vi "Load_Waveform.vi"(7 "Cmd":string="CWM", 8 "error in":errorcluster {"code" format="%.0x"}, 11 "RFSG_In":refnum<k15>="VST") -> (0 "error out":errorcluster, 3 "RFSG_Out":refnum<k15>="VST")   [LabVIEW 2014]
uses:
  <vilib>/RF Toolkits/LTE/SG/Support/Includes/nilte toolkit compatibility version.ctl
  <vilib>/RF Toolkits/WCDMA/Generation/Controls/niWCDMA SG Toolkit Compatibility Version.ctl
  <vilib>/RF Toolkits/GSM-EDGE/GSM/SG/Support/attribs.llb/Typedefs/niGSM SG Toolkit Compatibility Version.ctl
  <vilib>/RF Toolkits/GSM-EDGE/EDGE/SG/Support/attribs.llb/Typedefs/niEDGE SG Toolkit Compatibility Version.ctl
  <vilib>/RF Toolkits/LTE/SG/niLTE RFSG Create and Download Waveform (Single Antenna).vi
  <instrlib>/niRFSG/niRFSG.llb/niRFSG Write Arb Waveform (I-Q).vi
  <resource>/objmgr/niLTEGeneration.rc
  <resource>/objmgr/niWCDMAGeneration.rc
  <vilib>/RF Toolkits/GSM-EDGE/niGSMEDGE.lvlib
  <resource>/objmgr/niGSMGeneration.rc
  <resource>/objmgr/niEDGEGeneration.rc
panel:
  in  "Tab Control":T1(tab)=enum."CWM"
  out "Resource Element Map":dbl[][](graph)
  in  "PUSCH Modulation Scheme":i32(ring) items=["QPSK", "16-QAM", "64-QAM"]
  in  "System Bandwidth (Hz)":dbl(ring)=10000000.0 items=["1.4M"=1400000.0, "3M"=3000000.0, "5M"=5000000.0, "10M"=10000000.0, "15M"=15000000.0, "20M"=20000000.0]
  in  "Cyclic Prefix Mode":i32(ring) items=["Normal", "Extended"]
  in  "Cell ID":i32
  in  "Baseband Filter Enabled":i32(ring)=1 items=["False", "True"]
  in  "Duplex Mode":i32(ring)=1 items=["DL (FDD)", "UL (FDD)", "DL (TDD)", "UL (TDD)", "DL+UL (TDD)"]
  in  "UL/DL Configuration":i32(ring) items=["0", "1", "2", "3", "4", "5", "6"]
  in  "number of PUSCH resource blocks":i32=50
  in  "Carrier to Noise Ratio (dB)":dbl=50.0 format="%.2g"
  in  "AWGN Enabled":i32(ring) items=["False", "True"]
  in  "IQ Gain Imbalance (dB)":dbl format="%.2g"
  in  "Quadrature Skew (deg)":dbl format="%.2g"
  in  "Carrier Frequency Offset (Hz)":dbl format="%^.3e"
  in  "I DC Offset (%)":dbl format="%.2g"
  in  "Q DC Offset (%)":dbl format="%.2g"
  in  "Auto Headroom Enabled":i32(ring)=1 items=["False", "True"]
  in  "Headroom (dB)":dbl format="%.2g"
  out "Actual Headroom (dB)":dbl=5.0 format="%.2g"
  in  "Code Type":i32(ring) items=["Long", "Short"]
  in  "Code":i32
  in  "Uplink Test Case":enum32{"RMC1", "RMC2", "RMC3", "RMC4", "RMC5"}(ring)
  in  "All IQ Impairments Enabled":i32(ring)=1 items=["True"=1, "False"=0]
  in  "GSM_TSC":i32(ring) items=["TSC0", "TSC1", "TSC2", "TSC3", "TSC4", "TSC5", "TSC6", "TSC7"]
  in  "GSM_PN Order":i32=15
  in  "EDGE_TSC":i32(ring) items=["TSC0", "TSC1", "TSC2", "TSC3", "TSC4", "TSC5", "TSC6", "TSC7"]
  in  "EDGE_PN Order":i32=15
  in  "Wfm_Duration(s)":dbl=0.001
  in  "IQ_Rate":dbl=10000000.0 format="%#_6p"
  in  "Spacing Select":enum32{"Arbitrary Spacing", "Uniform Spacing"}(tab)=enum."Uniform Spacing"
  in  "Tone Parameters":T2(array[cluster])=[{"Offset (Hz)"=-100000.0, "Power Level (dBm)"=-20.0, "Initial Phase (degrees)"=0.0}, {"Offset (Hz)"=100000.0, "Power Level (dBm)"=-20.0, "Initial Phase (degrees)"=0.0}] {"Offset (Hz)" format="%#.3p"; "Initial Phase (degrees)" format="%.2f"; "Power Level (dBm)" format="%.2f"}
  in  "Mirror Image":bool
  in  "Number of Tones":i32=2
  in  "Power Level per Tone (dBm)":dbl=-10.0 format="%_3g"
  in  "Frequency Between Tones (Hz)":dbl=3000000.0 format="%#.3p"
  in  "Initial Phase (degrees)":dbl format="%_3g"
  out "Actual IQ Rate (S/s)":dbl=9999999.999999788 format="%#.3p"
  out "Power Level (dBm)":dbl=-6.9897000433601875 format="%#.3p"
  in  "Number of Samples":i32=100000
  in  "IQ Rate (S/sec)":dbl=10000000.0 format="%#.3p"
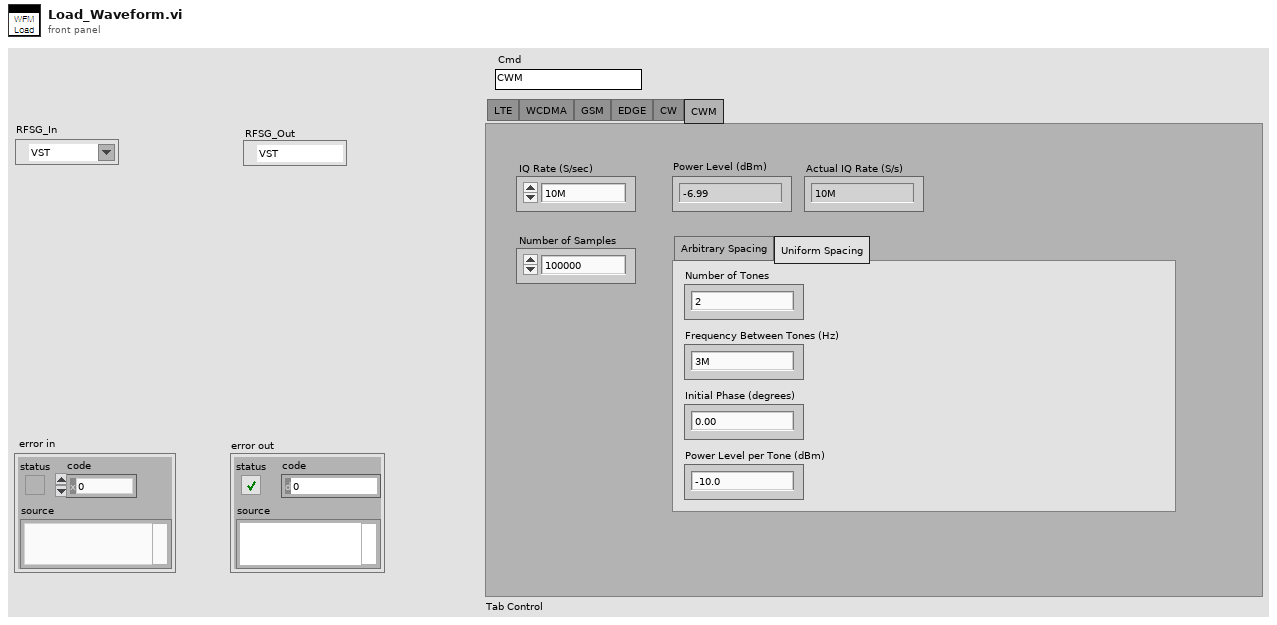
[diagram p1: front panel]
types:
  T1 = enum32{"LTE", "WCDMA", "GSM", "EDGE", "CW", "CWM"}
  T2 = cluster{"Offset (Hz)":dbl, "Power Level (dBm)":dbl, "Initial Phase (degrees)":dbl}[]
  T3 = typedef "nilte toolkit compatibility version.ctl" = i32
  T4 = typedef "nilte session.ctl" = refnum<k20>
  T5 = typedef "niWCDMA SG Toolkit Compatibility Version.ctl" = i32
  T6 = typedef "niWCDMA SG_Refnum.ctl" = refnum<k20>
  T7 = typedef "niGSMEDGE.lvlib/niGSM SG Toolkit Compatibility Version.ctl" = i32
  T8 = typedef "niGSMEDGE.lvlib/niGSM SG Refnum.ctl" = refnum<k20>
  T9 = typedef "niGSMEDGE.lvlib/niEDGE SG Toolkit Compatibility Version.ctl" = i32
  T10 = typedef "niGSMEDGE.lvlib/niEDGE SG Refnum.ctl" = refnum<k20>
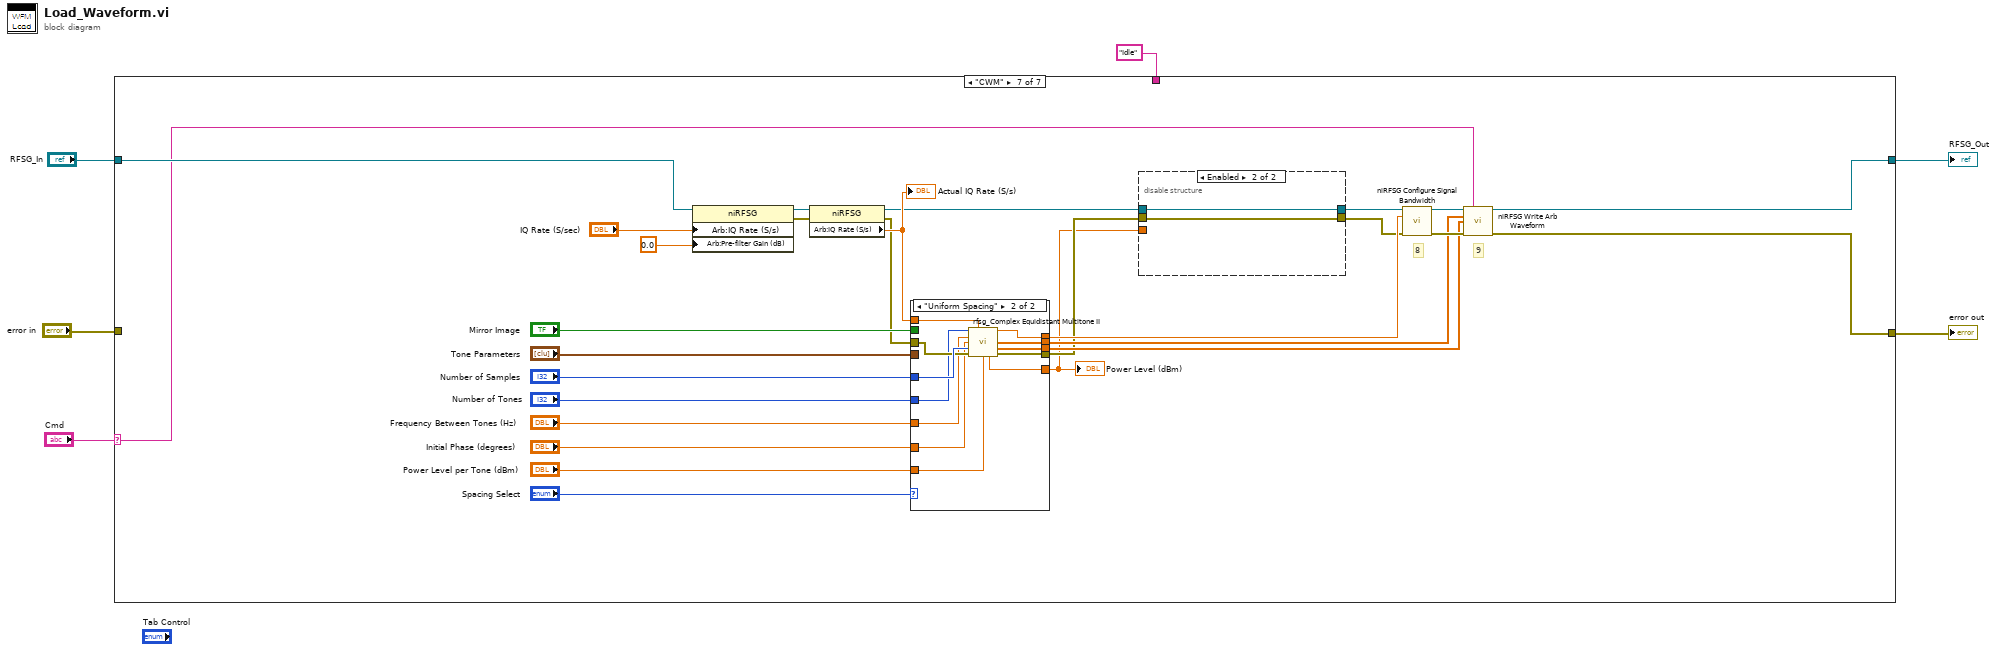
[diagram p0: block diagram]
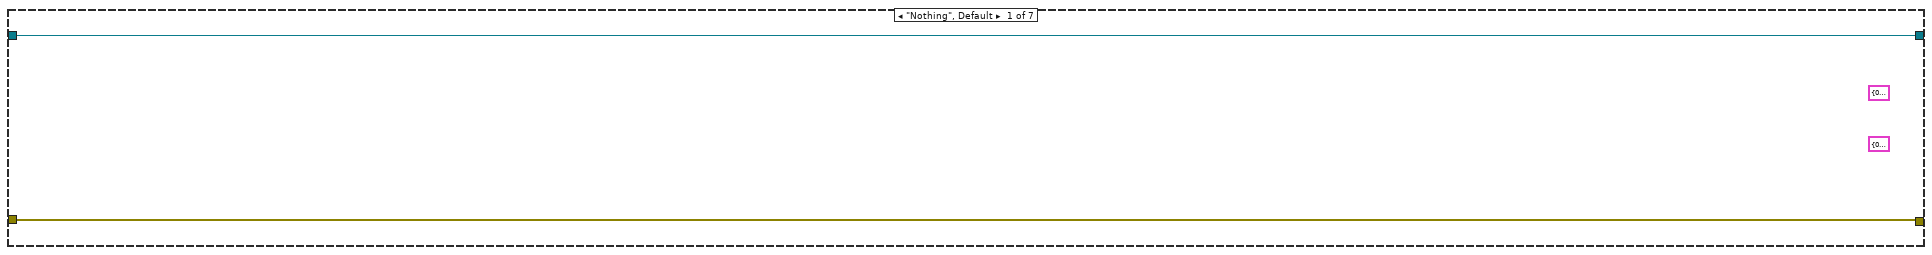
[diagram p2: hidden frame]
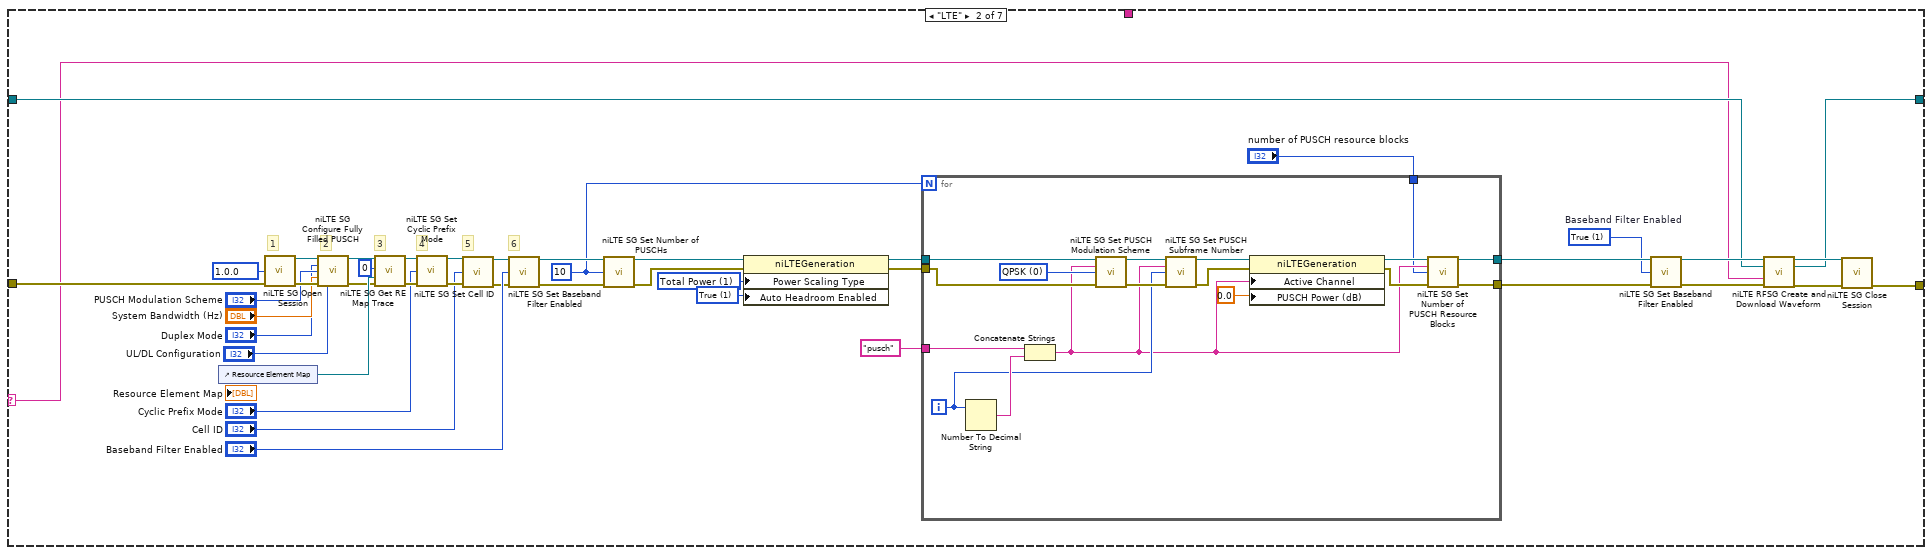
[diagram p3: hidden frame]
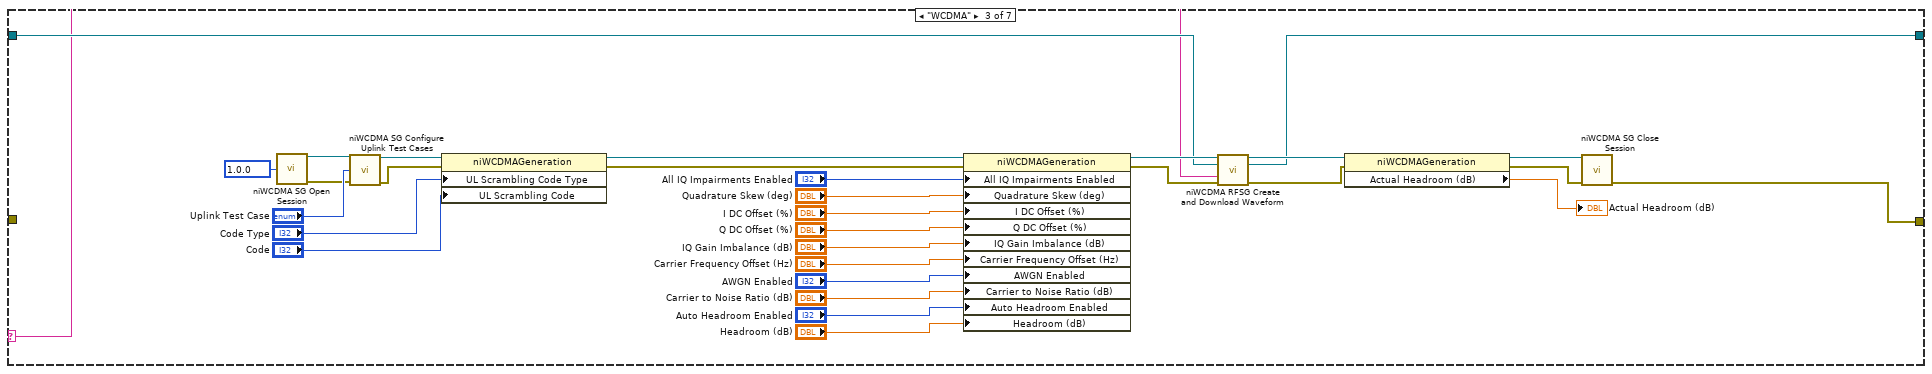
[diagram p4: hidden frame]
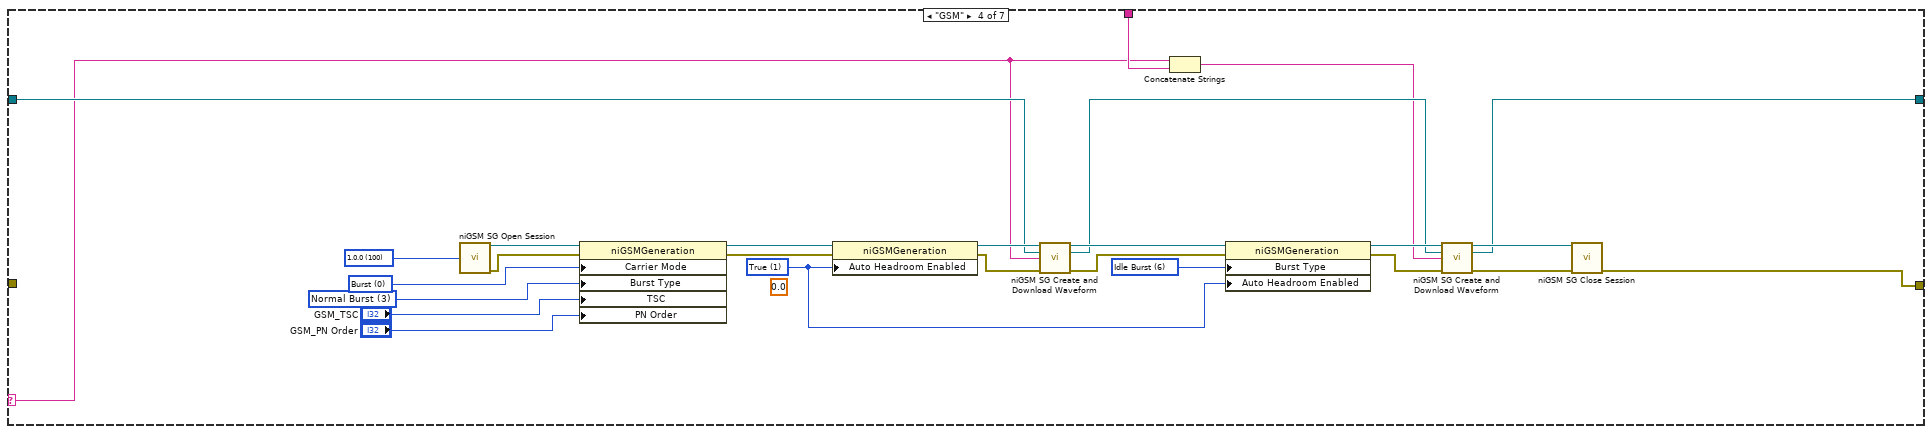
[diagram p5: hidden frame]
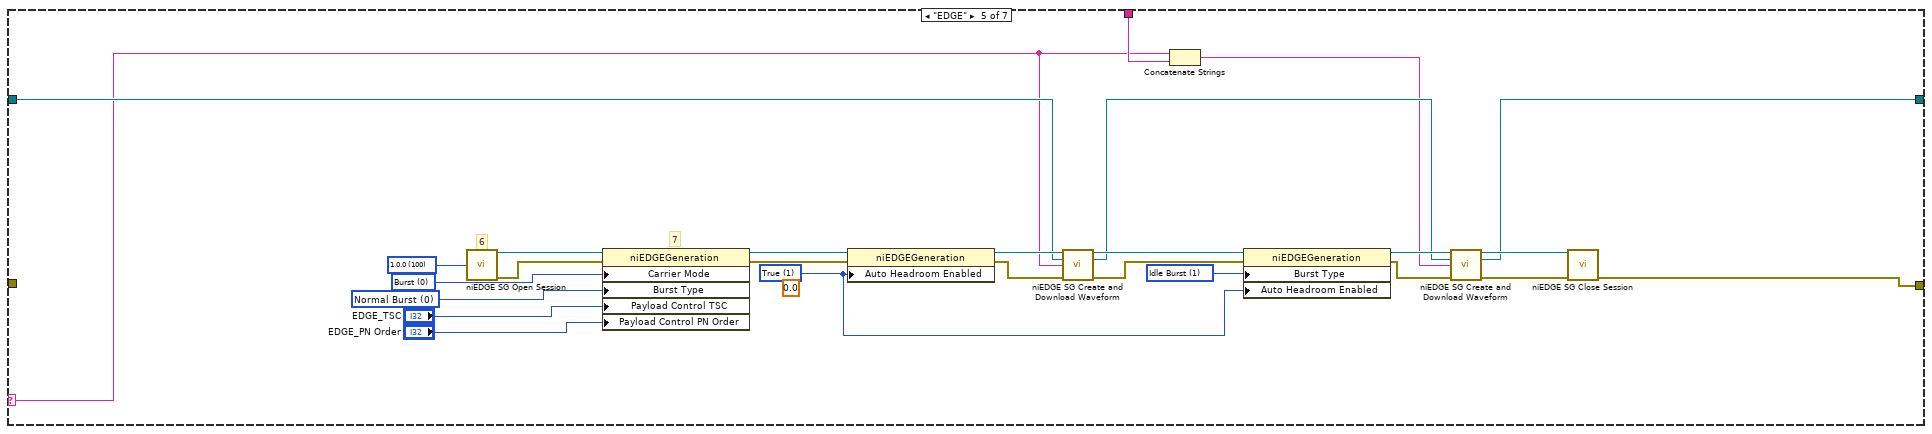
[diagram p6: hidden frame]
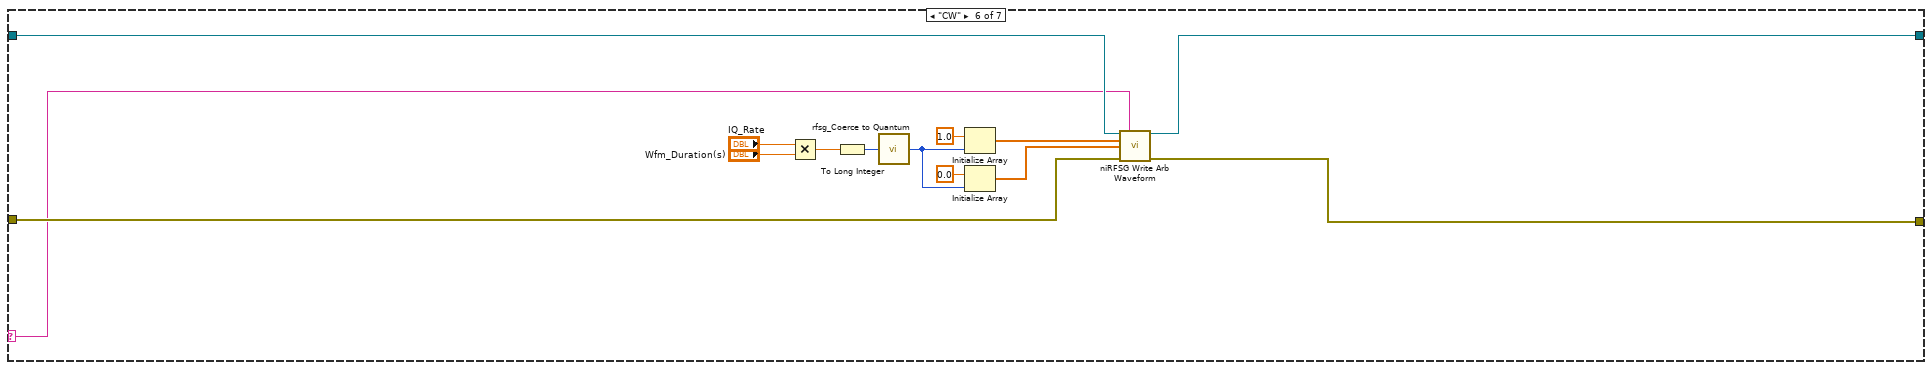
[diagram p7: hidden frame]
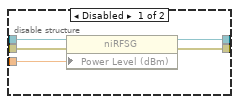
[diagram p8: hidden frame]
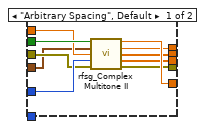
[diagram p9: hidden frame]
diagram:
  n1 = case shown="\"CWM\"" "Cmd" {
    selector: "Cmd" -> [_ w10 w69 w100 w126 w152 w167]
    tunnel: "RFSG_In" -> [w7 w14 w72 w110 w132 w156 w175]
    tunnel: [w7 w13 w71 w103 w130 w155 w169] -> w4
    tunnel: [w8 w12 w70 w109 w129 w153 w168] -> w3
    tunnel: "error in" -> [w8 w11 _ _ _ w154 _]
    tunnel: "Idle" ("Standard") -> [_ _ _ w102 w128 _ _]
    frame "Nothing", Default {
      (unwired) cluster{"t0":dbl, "dt":dbl, "Y":cdb[]} {"t0"=0.0, "dt"=0.0, "Y"=[]} ("complex signal out")
      (unwired) cluster{"t0":dbl, "dt":dbl, "Y":cdb[]} {"t0"=0.0, "dt"=0.0, "Y"=[]} ("complex signal out")
    }
    frame "LTE" {
      w9 = 1 items=["False", "True"]  # Baseband Filter Enabled
      w27 = 1 items=["Reference Signal Power", "Total Power"] ("Power Scaling Type")
      w26 = 1 items=["False", "True"] ("Auto Headroom Enabled")
      w25 = 10 ("number of PUSCHs")
      w51 = T3 10000 items=["1.0.0"=10000] ("toolkit compatibility version")
      # "6"
      # "5"
      # "4"
      # "3"
      # "2"
      # "1"
      n2 = control-ref of="Resource Element Map"() -> (w50:refnum<vi>)
      n3 = call <vilib>:"niLTE SG Open Session.vi"("toolkit compatibility version"=w51, "error in"=w11) -> ("niLTE SG session out"=w48:T4, "error out"=w47:errorcluster)  [unwired: 1 in, 11 out]
      n4 = call <vilib>:"niLTE SG Configure Fully Filled PUSCH.vi"("niLTE SG session"=w48, "duplex mode"="Duplex Mode", "PUSCH modulation scheme"="PUSCH Modulation Scheme", "system bandwidth (Hz)"="System Bandwidth (Hz)", "error in"=w47, "UL/DL configuration"="UL/DL Configuration") -> ("niLTE SG session out"=w44:T4, "error out"=w43:errorcluster)  [unwired: 8 out]
      n5 = call <vilib>:"niLTE SG Get RE Map Trace.vi"("niLTE SG session"=w44, "antenna port"=0, "intensity graph"=w50, "error in"=w43) -> ("niLTE SG session out"=w41:T4, "error out"=w40:errorcluster)  [unwired: 10 out]
      n6 = call <vilib>:"niLTE SG Set Cyclic Prefix Mode.vi"("niLTE SG session"=w41, "cyclic prefix mode"="Cyclic Prefix Mode", "error in"=w40) -> ("niLTE SG session out"=w46:T4, "error out"=w45:errorcluster)  [unwired: 11 out]
      n7 = call <vilib>:"niLTE SG Set Cell ID.vi"("niLTE SG session"=w46, "cell ID"="Cell ID", "error in"=w45) -> ("niLTE SG session out"=w35:T4, "error out"=w34:errorcluster)  [unwired: 11 out]
      n8 = call <vilib>:"niLTE SG Set Baseband Filter Enabled.vi"("niLTE SG session"=w35, "baseband filter enabled"="Baseband Filter Enabled", "error in"=w34) -> ("niLTE SG session out"=w31:T4, "error out"=w30:errorcluster)  [unwired: 11 out]
      n9 = call <vilib>:"niLTE SG Set Number of PUSCHs.vi"("niLTE SG session"=w31, "number of PUSCHs"=w25, "error in"=w30) -> ("niLTE SG session out"=w29:T4, "error out"=w28:errorcluster)  [unwired: 11 in]
      n10 = property class="niLTEGeneration"(reference=w29, error in=w28, "Power Scaling Type"=w27, "Auto Headroom Enabled"=w26) -> (reference out=w24:T4, error out=w23:errorcluster)
      n11 = for {
        N: w25 -> [_]
        tunnel: w24 -> [w66]
        tunnel: w23 -> [w65]
        tunnel: "pusch" -> [w68]
        tunnel: "number of PUSCH resource blocks" -> [w55]
        tunnel: [w54] -> w20
        tunnel: [w53] -> w19
        i -> [w61]
        w64 = 0 items=["QPSK", "16-QAM", "64-QAM"] ("PUSCH modulation scheme")
        n12 = Number To Decimal String(number=w61) -> (decimal integer string=w67:string)  [unwired: 1 in]
        n13 = Concatenate Strings(w68, w67) -> (w56:string)
        n14 = call <vilib>:"niLTE SG Set PUSCH Modulation Scheme.vi"("niLTE SG session"=w66, "active channel"=w56, "PUSCH modulation scheme"=w64, "error in"=w65) -> ("niLTE SG session out"=w63:T4, "error out"=w62:errorcluster)  [unwired: 10 in]
        n15 = call <vilib>:"niLTE SG Set PUSCH Subframe Number.vi"("niLTE SG session"=w63, "active channel"=w56, "PUSCH subframe number"=w61, "error in"=w62) -> ("niLTE SG session out"=w60:T4, "error out"=w59:errorcluster)  [unwired: 10 in]
        n16 = property class="niLTEGeneration"(reference=w60, error in=w59, "Active Channel"=w56, "PUSCH Power (dB)"=0.0) -> (reference out=w58:T4, error out=w57:errorcluster)
        n17 = call <vilib>:"niLTE SG Set Number of PUSCH Resource Blocks.vi"("niLTE SG session"=w58, "active channel"=w56, "number of PUSCH resource blocks"=w55, "error in"=w57) -> ("niLTE SG session out"=w54:T4, "error out"=w53:errorcluster)  [unwired: 10 in]
      }
      n18 = call <vilib>:"niLTE SG Set Baseband Filter Enabled.vi"("niLTE SG session"=w20, "baseband filter enabled"=w9, "error in"=w19) -> ("niLTE SG session out"=w17:T4, "error out"=w18:errorcluster)  [unwired: 11 out]
      n19 = call-poly <vilib>:"niLTE RFSG Create and Download Waveform.vi"("niLTE SG session"=w17, "instrument handle"=w14, "waveform name"=w10, "error in"=w18) -> ("niLTE SG session out"=w16:T4, "instrument handle out"=w13:refnum<k15>, "error out"=w15:errorcluster)  [unwired: 9 in]
      n20 = call <vilib>:"niLTE SG Close Session.vi"("niLTE SG session"=w16, "error in"=w15) -> ("error out"=w12:errorcluster)  [unwired: 13 out]
    }
    frame "WCDMA" {
      w77 = T5 10000 items=["1.0.0"=10000] ("toolkit compatibility version")
      n21 = call <vilib>:"niWCDMA SG Open Session.vi"("toolkit compatibility version"=w77) -> ("niWCDMA SG session out"=w81:T6, "error out"=w84:errorcluster)  [unwired: 2 in, 11 out]
      n22 = call <vilib>:"niWCDMA SG Configure Uplink Test Cases.vi"("niWCDMA SG session"=w81, "uplink test cases"="Uplink Test Case", "error in"=w84) -> ("niWCDMA SG session out"=w86:T6, "error out"=w87:errorcluster)  [unwired: 11 in]
      n23 = property class="niWCDMAGeneration"(reference=w86, error in=w87, "UL Scrambling Code Type"="Code Type", "UL Scrambling Code"="Code") -> (reference out=w88:T6, error out=w89:errorcluster)
      n24 = property class="niWCDMAGeneration"(reference=w88, error in=w89, "All IQ Impairments Enabled"="All IQ Impairments Enabled", "Quadrature Skew (deg)"="Quadrature Skew (deg)", "I DC Offset (%)"="I DC Offset (%)", "Q DC Offset (%)"="Q DC Offset (%)", "IQ Gain Imbalance (dB)"="IQ Gain Imbalance (dB)", "Carrier Frequency Offset (Hz)"="Carrier Frequency Offset (Hz)", "AWGN Enabled"="AWGN Enabled", "Carrier to Noise Ratio (dB)"="Carrier to Noise Ratio (dB)", "Auto Headroom Enabled"="Auto Headroom Enabled", "Headroom (dB)"="Headroom (dB)") -> (reference out=w75:T6, error out=w76:errorcluster)
      n25 = call <vilib>:"niWCDMA RFSG Create and Download Waveform.vi"("niWCDMA SG session"=w75, "instrument handle"=w72, "waveform name"=w69, "error in"=w76) -> ("niWCDMA SG session out"=w74:T6, "instrument handle out"=w71:refnum<k15>, "error out"=w73:errorcluster)  [unwired: 9 in]
      n26 = property class="niWCDMAGeneration"(reference=w74, error in=w73) -> (reference out=w78:T6, error out=w79:errorcluster, "Actual Headroom (dB)"=→"Actual Headroom (dB)":dbl)
      n27 = call <vilib>:"niWCDMA SG Close Session.vi"("niWCDMA SG session"=w78, "error in"=w79) -> ("error out"=w70:errorcluster)  [unwired: 13 out]
    }
    frame "GSM" {
      (unwired) 0.0 ("Headroom (dB)")
      w125 = 1 items=["False", "True"] ("Auto Headroom Enabled")
      w124 = 6 items=["Access Burst", "Dummy Burst", "Frequency Correction Burst", "Normal Burst", "Normal Burst CW", "Synchronization Burst", "Idle Burst"] ("Burst Type")
      w121 = T7 100 items=["1.0.0"=100] ("toolkit compatibility version")
      w120 = 0 items=["Burst", "Continuous"] ("Carrier Mode")
      w119 = 3 items=["Access Burst", "Dummy Burst", "Frequency Correction Burst", "Normal Burst", "Normal Burst CW", "Synchronization Burst", "Idle Burst"] ("Burst Type")
      n28 = call <vilib>:"niGSM SG Open Session.vi"("toolkit compatibility version"=w121) -> ("niGSM SG session out"=w118:T8, "error out"=w115:errorcluster)  [unwired: 2 in, 11 out]
      n29 = property class="niGSMGeneration"(reference=w118, error in=w115, "Carrier Mode"=w120, "Burst Type"=w119, "TSC"="GSM_TSC", "PN Order"="GSM_PN Order") -> (reference out=w122:T8, error out=w123:errorcluster)
      n30 = property class="niGSMGeneration"(reference=w122, error in=w123, "Auto Headroom Enabled"=w125) -> (reference out=w114:T8, error out=w112:errorcluster)
      n31 = call <vilib>:"niGSM SG Create and Download Waveform.vi"("niGSM SG session in"=w114, "instrument handle in"=w110, "waveform name"=w100, "error in"=w112) -> ("niGSM SG session out"=w113:T8, "instrument handle out"=w104:refnum<k15>, "error out"=w111:errorcluster)  [unwired: 9 in]
      n32 = Concatenate Strings(w100, w102) -> (w101:string)
      n33 = property class="niGSMGeneration"(reference=w113, error in=w111, "Burst Type"=w124, "Auto Headroom Enabled"=w125) -> (reference out=w108:T8, error out=w107:errorcluster)
      n34 = call <vilib>:"niGSM SG Create and Download Waveform.vi"("niGSM SG session in"=w108, "instrument handle in"=w104, "waveform name"=w101, "error in"=w107) -> ("niGSM SG session out"=w105:T8, "instrument handle out"=w103:refnum<k15>, "error out"=w106:errorcluster)  [unwired: 9 in]
      n35 = call <vilib>:"niGSM SG Close Session.vi"("niGSM SG session in"=w105, "error in"=w106) -> ("error out"=w109:errorcluster)  [unwired: 13 in]
    }
    frame "EDGE" {
      (unwired) 0.0 ("Headroom (dB)")
      w151 = 1 items=["False", "True"] ("Auto Headroom Enabled")
      w150 = 1 items=["Normal Burst"=0, "Higher Symbol Rate Burst"=2, "Idle Burst"=1] ("Burst Type")
      w147 = T9 100 items=["1.0.0"=100] ("toolkit compatibility version")
      w145 = 0 items=["Normal Burst", "Idle Burst"] ("Burst Type")
      w142 = 0 items=["Burst", "Continuous"] ("Carrier Mode")
      # "7"
      # "6"
      n36 = call <vilib>:"niEDGE SG Open Session.vi"("toolkit compatibility version"=w147) -> ("niEDGE SG session out"=w146:T10, "error out"=w141:errorcluster)  [unwired: 2 in, 11 out]
      n37 = property class="niEDGEGeneration"(reference=w146, error in=w141, "Carrier Mode"=w142, "Burst Type"=w145, "Payload Control TSC"="EDGE_TSC", "Payload Control PN Order"="EDGE_PN Order") -> (reference out=w149:T10, error out=w148:errorcluster)
      n38 = property class="niEDGEGeneration"(reference=w149, error in=w148, "Auto Headroom Enabled"=w151) -> (reference out=w140:T10, error out=w138:errorcluster)
      n39 = call <vilib>:"niEDGE SG Create and Download Waveform.vi"("niEDGE SG session in"=w140, "instrument handle in"=w132, "waveform name"=w126, "error in"=w138) -> ("niEDGE SG session out"=w139:T10, "instrument handle out"=w131:refnum<k15>, "error out"=w137:errorcluster)  [unwired: 9 in]
      n40 = Concatenate Strings(w126, w128) -> (w127:string)
      n41 = property class="niEDGEGeneration"(reference=w139, error in=w137, "Burst Type"=w150, "Auto Headroom Enabled"=w151) -> (reference out=w136:T10, error out=w135:errorcluster)
      n42 = call <vilib>:"niEDGE SG Create and Download Waveform.vi"("niEDGE SG session in"=w136, "instrument handle in"=w131, "waveform name"=w127, "error in"=w135) -> ("niEDGE SG session out"=w133:T10, "instrument handle out"=w130:refnum<k15>, "error out"=w134:errorcluster)  [unwired: 9 in]
      n43 = call <vilib>:"niEDGE SG Close Session.vi"("niEDGE SG session in"=w133, "error in"=w134) -> ("error out"=w129:errorcluster)  [unwired: 13 in]
    }
    frame "CW" {
      n44 = Multiply(x="IQ_Rate", y="Wfm_Duration(s)") -> (x*y=w163:dbl)
      n45 = To Long Integer(number=w163) -> (32bit integer=w161:i32)
      n46 = call <instrlib>:"rfsg_Coerce to Quantum.vi"("samples"=w161) -> ("coerced to quantum"=w162:i32)  [unwired: 3 in]
      n47 = Initialize Array(1.0 ("element"), w162) -> (w157:dbl[])
      n48 = Initialize Array(0.0 ("element"), w162) -> (w158:dbl[])
      n49 = call-poly <instrlib>:"niRFSG Write Arb Waveform.vi"("instrument handle"=w156, "name"=w152, "I Data"=w157, "Q Data"=w158, "error in"=w154) -> ("instrument handle out"=w155:refnum<k15>, "error out"=w153:errorcluster)  [unwired: 9 in]
    }
    frame "CWM" {
      # "9"
      # "8"
      n50 = property class="niRFSG"(reference=w175, "Arb:IQ Rate (S/s)"="IQ Rate (S/sec)", "Arb:Pre-filter Gain (dB)"=0.0 ("RF:Advanced:AWG:DUC Pre-filter Gain (dB)")) -> (reference out=w192:refnum<k15>, error out=w191:errorcluster)  [unwired: 1 in]
      n51 = property class="niRFSG"(reference=w192, error in=w191) -> (reference out=w170:refnum<k15>, error out=w180:errorcluster, "Arb:IQ Rate (S/s)"=w182:dbl)
      "Actual IQ Rate (S/s)" <- w182
      n52 = case shown="\"Uniform Spacing\"" "Spacing Select" {
        tunnel: "Mirror Image" -> [w210 _]
        tunnel: "Tone Parameters" -> [w201 _]
        tunnel: "Number of Samples" -> [w209 w217]
        tunnel: [w208 w218] -> w171
        tunnel: [w207 w222] -> w185
        tunnel: [w206 w219] -> w172
        tunnel: [w205 w221] -> w184
        tunnel: [w204 w220] -> w183
        tunnel: w182 -> [w203 w215]
        tunnel: w180 -> [w202 w216]
        tunnel: "Number of Tones" -> [_ w214]
        tunnel: "Frequency Between Tones (Hz)" -> [_ w213]
        tunnel: "Initial Phase (degrees)" -> [_ w212]
        tunnel: "Power Level per Tone (dBm)" -> [_ w211]
        frame "Arbitrary Spacing", Default {
          n53 = call <instrlib>:"rfsg_Complex Multitone II.vi"("Mirror Image"=w210, "Tone Parameters"=w201, "Sample Rate (S/s)"=w203, "Samples"=w209, "Error In"=w202) -> ("Signal Power Level (dBm)"=w208:dbl, "Signal Bandwidth (Hz)"=w207:dbl, "I Data"=w205:dbl[], "Q Data"=w204:dbl[], "Error Out"=w206:errorcluster)  [unwired: 6 in]
        }
        frame "Uniform Spacing" {
          n54 = call <instrlib>:"rfsg_Complex Equidistant Multitone II.vi"("Number of Tones"=w214, "Sample Rate (Hz)"=w215, "Desired Frequency Between Tones (Hz)"=w213, "Initial Phase (degrees)"=w212, "Max. Number of Samples"=w217, "Error In"=w216, "Power Level per Tone (dBm)"=w211) -> ("Signal Bandwidth"=w222:dbl, "I Data"=w221:dbl[], "Q Data"=w220:dbl[], "Signal Power Level (dBm)"=w218:dbl, "Error Out"=w219:errorcluster)  [unwired: 3 in, 1 out]
        }
      }
      "Power Level (dBm)" <- w171
      n55 = disable-structure shown="Enabled" {
        disable-tunnel: [w198 w200] -> w174
        disable-tunnel: [w197 w199] -> w173
        disable-tunnel: w172 -> [w196 w199]
        disable-tunnel: w171 -> [w195 _]
        disable-tunnel: w170 -> [w194 w200]
        frame Disabled {
          n56 = property class="niRFSG"(reference=w194, error in=w196, "Power Level (dBm)"=w195) -> (reference out=w198:refnum<k15>, error out=w197:errorcluster)
        }
        frame Enabled {
        }
      }
      n57 = call <instrlib>:"niRFSG Configure Signal Bandwidth.vi"("instrument handle"=w174, "signal bandwidth (Hz)"=w185, "error in"=w173) -> ("instrument handle out"=w193:refnum<k15>, "error out"=w190:errorcluster)  [unwired: 11 in]
      n58 = call-poly <instrlib>:"niRFSG Write Arb Waveform.vi"("instrument handle"=w193, "name"=w167, "I Data"=w184, "Q Data"=w183, "error in"=w190) -> ("instrument handle out"=w169:refnum<k15>, "error out"=w168:errorcluster)  [unwired: 9 in]
    }
  }
  "RFSG_Out" <- w4
  "error out" <- w3
